vi "Filter Out Infinite Indices.vi"(10 "Closest Point Indices in":i32[][](array[numeric]), 11 "Infinite Regions":set{i32}(c389)) -> (3 "Closest Point Indices out":i32[][](array[numeric]))   [LabVIEW 2019]
doc: "Filter out infinite indices"
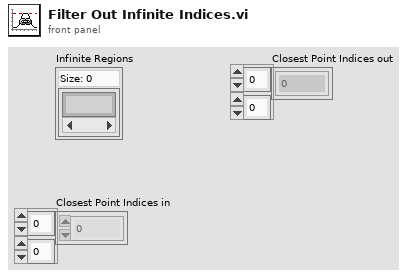
[diagram p1: front panel]
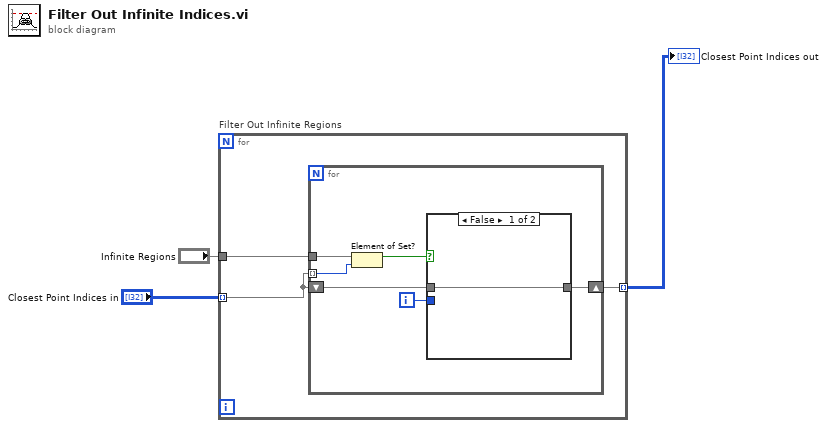
[diagram p0: block diagram]
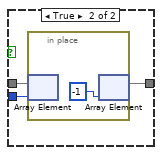
[diagram p2: hidden frame]
diagram:
  n1 = for "Filter Out Infinite Regions" {
    tunnel: "Closest Point Indices in" -> [w6] mode=indexing
    tunnel: [w5] -> w3 mode=indexing
    tunnel: "Infinite Regions" -> [w4]
    n2 = for {
      tunnel: w6 -> [w8] mode=indexing
      shift-right: [w10] -> w5
      shift-left: w6 -> [w12]
      tunnel: w4 -> [w9]
      i -> [w11]
      n3 = Element of Set?(10:w8, 11:w9) -> (3:w7:bool)
      n4 = case shown="False" w7 {
        tunnel: w12 -> [w13 w16]
        tunnel: w11 -> [_ w15]
        tunnel: [w13 w14] -> w10
        frame False {
        }
        frame True {
          n5 = in-place {
            n6 = in-place-array #1(w16, w15) -> ()  [unwired: 1 out]
            n7 = in-place-array #1(-1 ("f")) -> (w14:i32[])  [unwired: 1 out]
          }
        }
      }
    }
  }
  "Closest Point Indices out" <- w3
